vi "Tag Example.vi"() -> ()   [LabVIEW 2016]
uses:
  <vilib>/TagLibrary/Create Tag (Int).vi
  <vilib>/TagLibrary/Write (Int).vi
  <vilib>/TagLibrary/Close Tag (Single).vi
  <vilib>/TagLibrary/TagLibrary.lvlib
panel:
  in  "int":i32 caption="integer"
  in  "tag path":string="foo.bar"
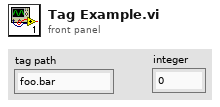
[diagram p1: front panel]
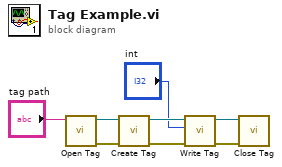
[diagram p0: block diagram]
diagram:
  n1 = call <vilib>:"Open Tag.vi"("tag path"="tag path") -> ("error out"=w1:errorcluster, "tag reference out"=w2:refnum<k21>)  [unwired: 9 in]
  n2 = call-poly <vilib>:"Create Tag.vi"("error in (no error)"=w1, "tag reference in"=w2) -> ("error out"=w4:errorcluster, "tag reference out"=w5:refnum<k21>)  [unwired: 8 in]
  n3 = call-poly <vilib>:"Write Tag.vi"("error in (no error)"=w4, "int"="int", "tag reference in"=w5) -> ("error out"=w7:errorcluster, "tag reference out"=w6:refnum<k21>)  [unwired: 7 in]
  n4 = call-poly <vilib>:"Close Tag.vi"("error in (no error)"=w7, "tag reference"=w6) -> ()  [unwired: 9 in, 1 out]
